vi "DAQ_SerialNumber.vi"(8 "error in (no error)":errorcluster, 11 "ActiveDev":tag="Dev1") -> (0 "error out":errorcluster, 3 "DevSerialNum":string)   [LabVIEW 2015]
uses:
  <resource>/objmgr/daqmx.rc
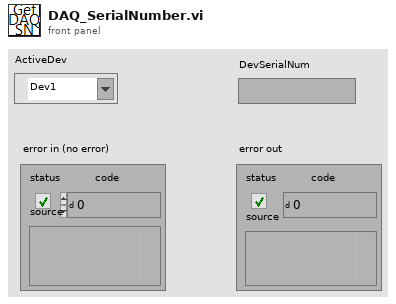
[diagram p1: front panel]
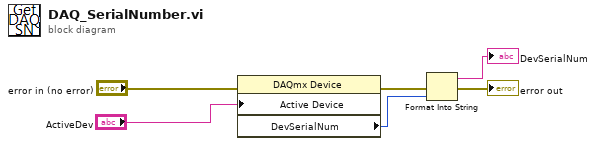
[diagram p0: block diagram]
diagram:
  n1 = property class="DAQmx Device"(error in="error in (no error)", "Active Device"="ActiveDev") -> (error out=w3:errorcluster, "DevSerialNum"=w5:u32)  [unwired: 1 in, 1 out]
  n2 = Format Into String(error in=w3, w5) -> (resulting string=→"DevSerialNum":string, error out=→"error out":errorcluster)  [unwired: 2 in]
